vi "BinaryTest.vi"() -> ()   [LabVIEW 2011]
panel:
  in  "Stop Button":bool
  out "Number":u32
  in  "Binary Array":bool[](array[boolean])
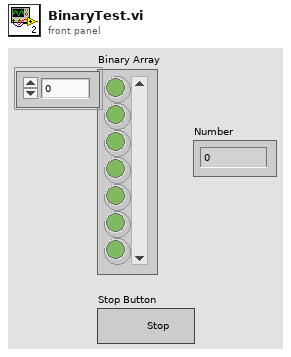
[diagram p1: front panel]
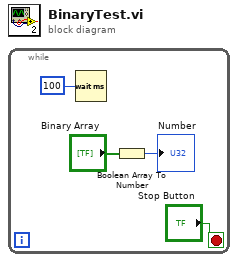
[diagram p0: block diagram]
diagram:
  n1 = while {
    stop <- "Stop Button" stop-if-true
    n2 = Wait (ms)(milliseconds to wait=u32 100) -> ()  [unwired: 1 out]
    n3 = Boolean Array To Number(Boolean array="Binary Array") -> (number=→"Number":u32)
  }
